vi "VNA.vi"() -> ()   [LabVIEW 2022 SP3]
uses:
  <vilib>/Utility/file.llb/Write Delimited Spreadsheet (DBL).vi
  Agilent ENA Series/Agilent ENA Series.lvlib
panel:
  in  "wait time (ms)":dbl
  in  "Smoothing State (F: Off)":bool
  in  "IF Bandwidth (100000.0)":dbl=1000.0 format="%^.1e"
  in  "Average Factor (16)":i32=16
  in  "Averaging State (F: Off)":bool
  in  "Continuous Sweep (T: Enable)":bool=TRUE
  in  "Point Trigger (F: Disable)":bool
  in  "Trigger Source":u16(ring) items=["Internal", "External", "Manual", "BUS"]
  in  "Stop (MHz)":dbl format="%^.2e"
  in  "Start (Mhz)":dbl=1.0 format="%^.2e"
  in  "Number of Measurement Points":i32=1001
  in  "Power Level (dBm)":dbl=-5.0 format="%^.2g"
  in  "file path (dialog if empty)":path
  in  "Measurement Parameters":u16(ring)=1 items=["S11", "S21", "S31", "S41", "S12", "S22", "S32", "S42", "S13", "S23", "S33", "S43", "S14", "S24", "S34", "S44", "A", "B", "C", "D", "R1", "R2", "R3", "R4"]
  out "Waveform Graph":dbl[](graph)
  in  "Safe Mode Maximum Power Level (30)":dbl=30.0
  in  "Safe Mode Minimum Power Level (-200)":dbl=-200.0
  in  "Tolerance Level (5)":dbl=5.0
  in  "Power Level Offset (0)":dbl
  in  "Port ( 1)":i32=1
  in  "Channel (1)":i32=1
  in  "Enable Safe Mode (T: Enabled)":bool=TRUE
  in  "Enable Receiver Leveling (T: Enabled)":bool=TRUE
  in  "Reset? (T: Yes)":bool=TRUE
  in  "ID Query? (T: Yes)":bool=TRUE
  in  "VISA resource name":refnum<visa-resource-name>="E5061A"
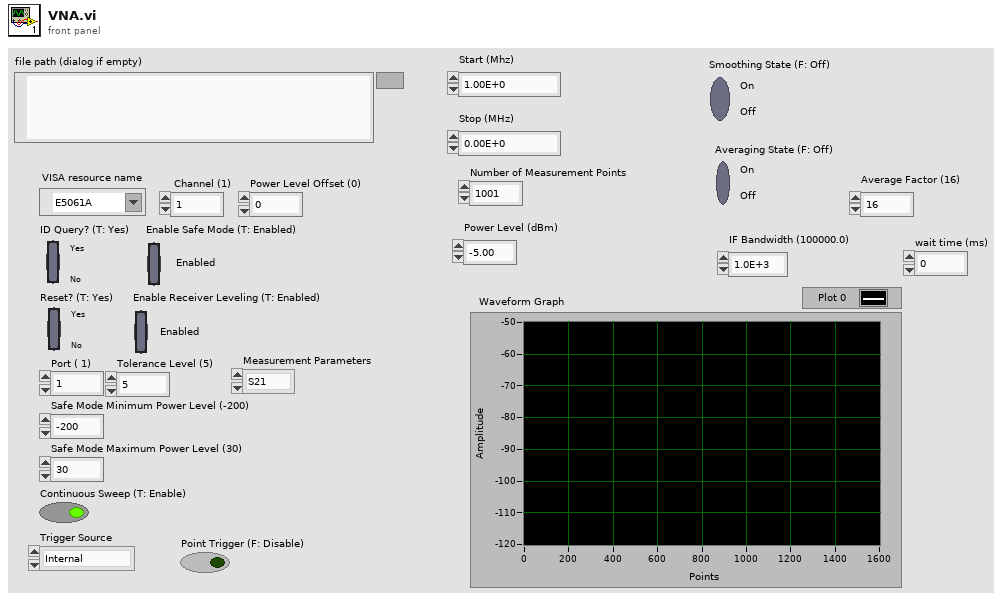
[diagram p1: front panel]
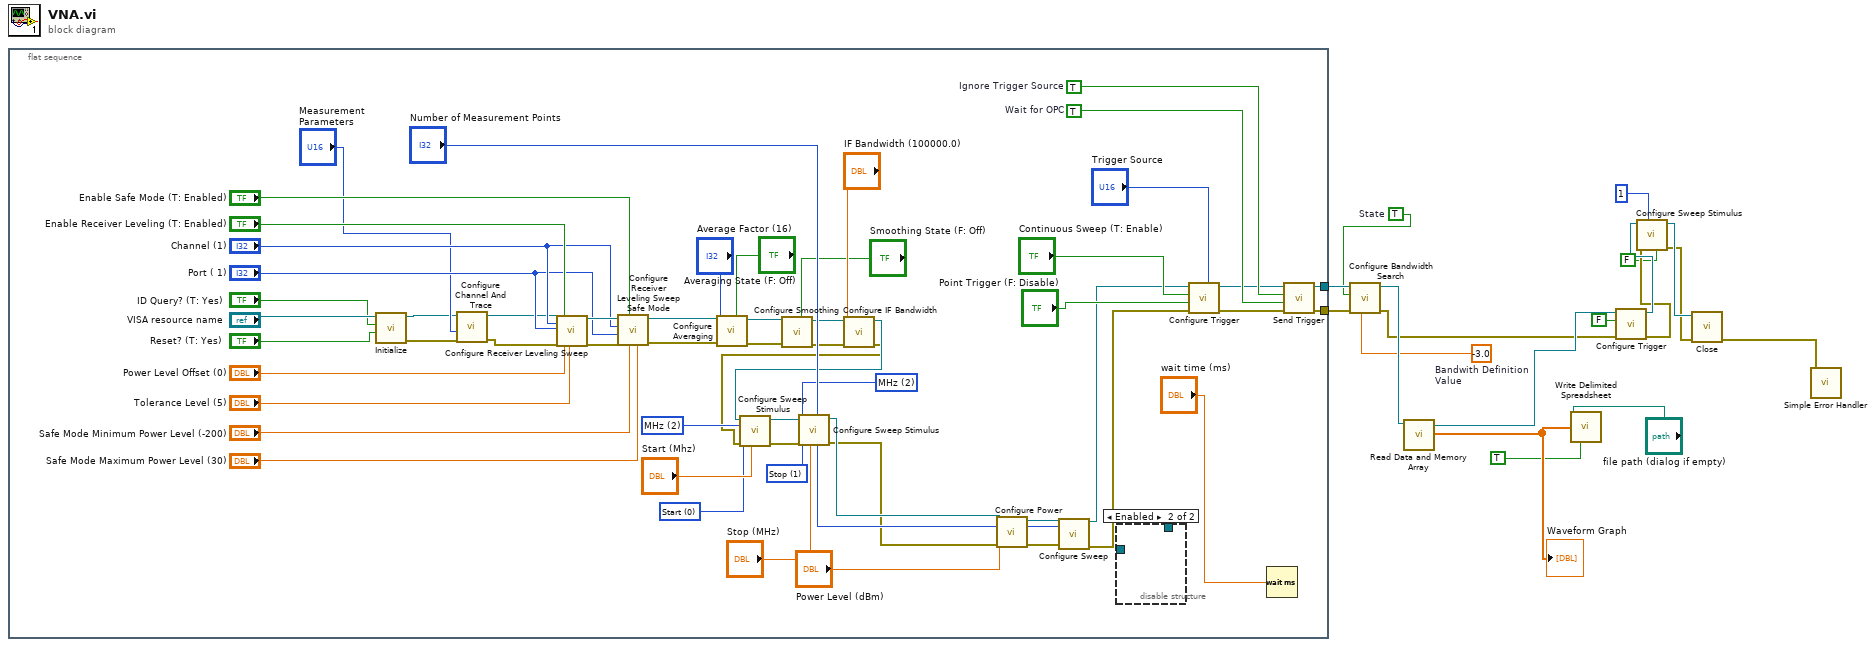
[diagram p0: block diagram]
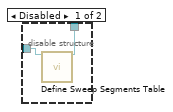
[diagram p2: hidden frame]
diagram:
  w9 = TRUE  # State
  w10 = -3.0  # Bandwith Definition Value
  n1 = flat-sequence {
    tunnel: [w72] -> w11
    tunnel: [w20] -> w8
    frame #0 {
      w47 = u16 2 items=["Hz", "kHz", "MHz", "GHz", "dBm", "s", "V"] ("Unit (0: Hz)")
      w48 = u16 2 items=["Hz", "kHz", "MHz", "GHz", "dBm", "s", "V"] ("Unit (0: Hz)")
      w49 = u16 1 items=["Start", "Stop", "Center", "Span"] ("Stimulus (0: Start)")
      w50 = u16 0 items=["Start", "Stop", "Center", "Span"] ("Stimulus (0: Start)")
      w73 = TRUE  # Wait for OPC
      w74 = TRUE  # Ignore Trigger Source
      n2 = call "Initialize.vi"("Reset? (T: Yes)"="Reset? (T: Yes)", "ID Query? (T: Yes)"="ID Query? (T: Yes)", "VISA resource name"="VISA resource name") -> ("error out"=w32:errorcluster, "VISA resource name out"=w36:refnum<visa-resource-name>)  [unwired: 7 in]
      n3 = call "Configure Channel And Trace.vi"("error in (no error)"=w32, "Measurement Parameters (0: S11)"="Measurement Parameters", "VISA resource name"=w36) -> ("error out"=w31:errorcluster, "VISA resource name out"=w35:refnum<visa-resource-name>)  [unwired: 7 in]
      n4 = call "Configure Receiver Leveling Sweep.vi"("VISA resource name"=w35, "Channel (1)"="Channel (1)", "Port ( 1)"="Port ( 1)", "error in (no error)"=w31, "Enable Receiver Leveling (F: Disabled)"="Enable Receiver Leveling (T: Enabled)", "Power Level Offset (0)"="Power Level Offset (0)", "Tolerance Level (5)"="Tolerance Level (5)") -> ("VISA resource name out"=w67:refnum<visa-resource-name>, "error out"=w30:errorcluster)  [unwired: 11 in]
      n5 = call "Configure Receiver Leveling Sweep Safe Mode.vi"("Safe Mode Maximum Power Level (30)"="Safe Mode Maximum Power Level (30)", "Safe Mode Minimum Power Level (-200)"="Safe Mode Minimum Power Level (-200)", "Enable Safe Mode (F: Disabled)"="Enable Safe Mode (T: Enabled)", "error in (no error)"=w30, "Port ( 1)"="Port ( 1)", "Channel (1)"="Channel (1)", "VISA resource name"=w67) -> ("error out"=w29:errorcluster, "VISA resource name out"=w34:refnum<visa-resource-name>)  [unwired: 3 in]
      n6 = call "Configure Averaging.vi"("Averaging State (F: Off)"="Averaging State (F: Off)", "error in (no error)"=w29, "Factor (16)"="Average Factor (16)", "VISA resource name"=w34) -> ("error out"=w28:errorcluster, "VISA resource name out"=w43:refnum<visa-resource-name>)  [unwired: 6 in]
      n7 = call "Configure Smoothing.vi"("Smoothing State (F: Off)"="Smoothing State (F: Off)", "error in (no error)"=w28, "VISA resource name"=w43) -> ("error out"=w27:errorcluster, "VISA resource name out"=w42:refnum<visa-resource-name>)  [unwired: 7 in]
      n8 = call "Configure IF Bandwidth.vi"("error in (no error)"=w27, "IF Bandwidth (100000.0)"="IF Bandwidth (100000.0)", "VISA resource name"=w42) -> ("error out"=w26:errorcluster, "VISA resource name out"=w41:refnum<visa-resource-name>)  [unwired: 7 in]
      n9 = call "Configure Sweep Stimulus.vi"("Parameter (0.0)"="Start (Mhz)", "error in (no error)"=w26, "Stimulus (0: Start)"=w50, "Unit (0: Hz)"=w48, "VISA resource name"=w41) -> ("error out"=w25:errorcluster, "VISA resource name out"=w54:refnum<visa-resource-name>)  [unwired: 5 in]
      n10 = call "Configure Sweep Stimulus.vi"("Parameter (0.0)"="Stop (MHz)", "error in (no error)"=w25, "Stimulus (0: Start)"=w49, "Unit (0: Hz)"=w47, "VISA resource name"=w54) -> ("error out"=w24:errorcluster, "VISA resource name out"=w53:refnum<visa-resource-name>)  [unwired: 5 in]
      n11 = call "Configure Power.vi"("VISA resource name"=w53, "Power Level (0.0)"="Power Level (dBm)", "error in (no error)"=w24) -> ("VISA resource name out"=w56:refnum<visa-resource-name>, "error out"=w23:errorcluster)  [unwired: 11 in]
      n12 = call "Configure Sweep.vi"("VISA resource name"=w56, "Number of Measurement Points (201)"="Number of Measurement Points", "error in (no error)"=w23) -> ("VISA resource name out"=w33:refnum<visa-resource-name>, "error out"=w22:errorcluster)  [unwired: 11 in]
      n13 = disable-structure shown="Enabled" {
        disable-tunnel: _ -> [w76 _]
        disable-tunnel: [w75 _] -> _
        frame Disabled {
          n14 = call <instrlib>:"Define Sweep Segments Table.vi"("VISA resource name"=w76) -> ("VISA resource name out"=w75:refnum<visa-resource-name>)  [unwired: 17 in, 1 out]
        }
        frame Enabled {
        }
      }
      n15 = call "Configure Trigger.vi"("Trigger Source (0: Internal)"="Trigger Source", "error in (no error)"=w22, "Point Trigger (F: Disable)"="Point Trigger (F: Disable)", "Continuous Sweep (T: Enable)"="Continuous Sweep (T: Enable)", "VISA resource name"=w33) -> ("error out"=w21:errorcluster, "VISA resource name out"=w68:refnum<visa-resource-name>)  [unwired: 5 in]
      n16 = Wait (ms)(milliseconds to wait="wait time (ms)") -> ()  [unwired: 1 out]
      n17 = call "Send Trigger.vi"("error in (no error)"=w21, "Wait for OPC (F: Do not Wait)"=w73, "Ignore Trigger Source (F: Do not Ignore)"=w74, "VISA resource name"=w68) -> ("error out"=w20:errorcluster, "VISA resource name out"=w72:refnum<visa-resource-name>)  [unwired: 6 in]
    }
  }
  n18 = call "Configure Bandwidth Search.vi"("Bandwidth Definition Value (-3.0)"=w10, "error in (no error)"=w8, "Result Display State (F: Disable)"=w9, "VISA resource name"=w11) -> ("error out"=w7:errorcluster, "VISA resource name out"=w12:refnum<visa-resource-name>)  [unwired: 6 in]
  n19 = call "Read Data and Memory Array.vi"("VISA resource name"=w12) -> ("Primary / Real"=w17:dbl[], "VISA resource name out"=w14:refnum<visa-resource-name>)  [unwired: 7 in, 2 out]
  "Waveform Graph" <- w17
  n20 = call-poly <vilib>:"Write Delimited Spreadsheet.vi"("file path (dialog if empty)"="file path (dialog if empty)", "1D data"=w17, "transpose? (no:F)"=TRUE) -> ()  [unwired: 11 in, 2 out]
  n21 = call "Configure Trigger.vi"("error in (no error)"=w7, "Continuous Sweep (T: Enable)"=FALSE, "VISA resource name"=w14) -> ("error out"=w4:errorcluster, "VISA resource name out"=w6:refnum<visa-resource-name>)  [unwired: 7 in]
  n22 = call "Configure Sweep Stimulus.vi"("Signal Output (T: On)"=FALSE, "Channel (1)"=1, "error in (no error)"=w4, "VISA resource name"=w6) -> ("error out"=w3:errorcluster, "VISA resource name out"=w5:refnum<visa-resource-name>)  [unwired: 6 in]
  n23 = call "Close.vi"("error in (no error)"=w3, "VISA resource name"=w5) -> ("error out"=w18:errorcluster)  [unwired: 9 in]
  n24 = call <vilib>:"Simple Error Handler.vi"("error in (no error)"=w18) -> ()  [unwired: 4 in, 5 out]
